vi "Set Display Reading Format.vi"(0 "VISA resource name":refnum<visa-resource-name>, 5 "Reading Format":u16(ring) items=["Exponent", "Prefix"], 11 "error in (no error)":errorcluster) -> (4 "VISA resource name out":refnum<visa-resource-name>, 15 "error out":errorcluster)   [LabVIEW 2023, in "Keithley DMM6500 DAQ6500 Series.lvlib"]
doc: "Sets the format (Exponent or Engineering notation/unit prefix) that is used to display measurement readings on the front-panel display of the instrument."
uses:
  <instrlib>/Keithley DMM6500 DAQ6500 Series/Keithley DMM6500 DAQ6500 Series.lvlib
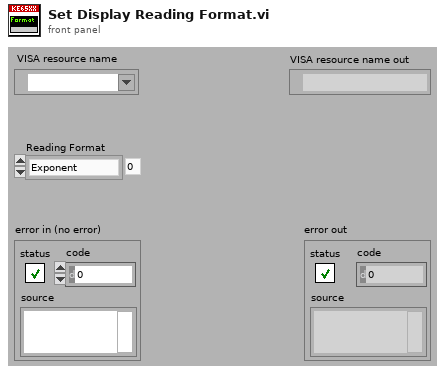
[diagram p1: front panel]
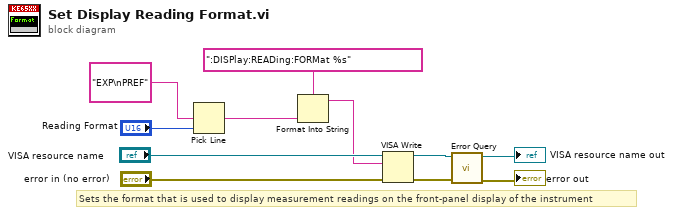
[diagram p0: block diagram]
diagram:
  # "Sets the format that is used to display measurement readings on the front-panel display of the instrument"
  n1 = Pick Line(multi-line string="EXP\nPREF", line index="Reading Format") -> (output string=w6:string)  [unwired: 1 in]
  n2 = Format Into String(format string=":DISPlay:READing:FORMat %s", w6) -> (resulting string=w5:string)  [unwired: 2 in, 1 out]
  n3 = VISA Write(VISA resource name="VISA resource name", write buffer=w5, error in (no error)="error in (no error)") -> (VISA resource name out=w4:refnum<visa-resource-name>, error out=w3:errorcluster)  [unwired: 1 out]
  n4 = call <instrlib>:"Error Query.vi"("error in (no error)"=w3, "VISA resource name"=w4) -> ("error out"=→"error out":errorcluster, "VISA resource name out"=→"VISA resource name out":refnum<visa-resource-name>)  [unwired: 6 in, 2 out]
